vi "ArmTest_LE_and_XZ-AUTO.vi"() -> ()   [LabVIEW 2023]
doc: "Auto test program that coverts RLE to XYZ then to XYZ to RLE"
uses:
  <vilib>/Rock Robotics/WPI/ThirdParty/JAS_Junk/TrajLib/Trajectory_Library.lvlib
panel:
  out "Passed":bool
  out "Extend 2":dbl
  out "Lift 2":dbl
  out "z":dbl
  out "x":dbl
  out "Lift":dbl
  out "Extend":dbl
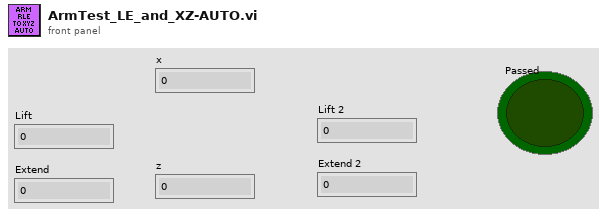
[diagram p1: front panel]
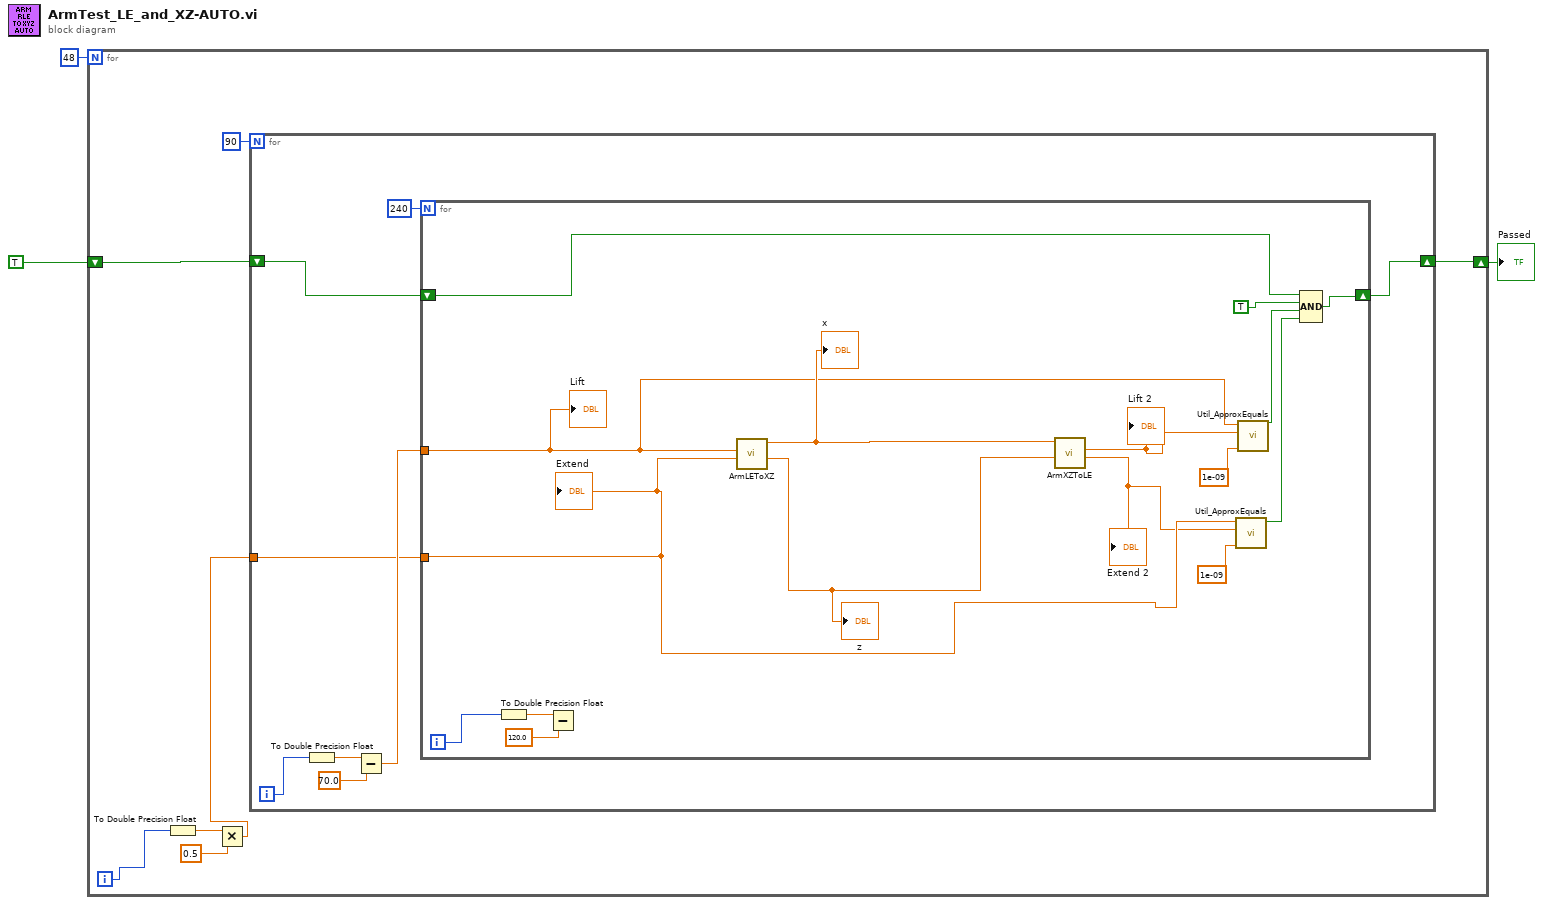
[diagram p0: block diagram]
diagram:
  n1 = for {
    N: 48 -> [_]
    shift-right: [w4] -> w1
    shift-left: TRUE -> [w5]
    i -> [w7]
    n2 = To Double Precision Float(number=w7) -> (double precision float=w9:dbl)
    n3 = Multiply(x=w9, y=0.5) -> (x*y=w6:dbl)
    n4 = for {
      N: 90 -> [_]
      tunnel: w6 -> [w13]
      shift-right: [w11] -> w4
      shift-left: w5 -> [w12]
      i -> [w15]
      n5 = To Double Precision Float(number=w15) -> (double precision float=w17:dbl)
      n6 = Subtract(x=w17, y=70.0) -> (x-y=w14:dbl)
      n7 = for {
        N: 240 -> [_]
        tunnel: w14 -> [w27]
        tunnel: w13 -> [w25]
        shift-right: [w20] -> w11
        shift-left: w12 -> [w23]
        i -> [w32]
        n8 = To Double Precision Float(number=w32) -> (double precision float=w31:dbl)
        n9 = Subtract(x=w31, y=120.0) -> ()  [unwired: 1 out]
        n10 = call "ArmLEToXZ.vi"("Extend"=w25, "Lift"=w27) -> ("z"=w33:dbl, "x"=w34:dbl)  [unwired: 8 in]
        "x" <- w34
        "z" <- w33
        n11 = call "ArmXZToLE.vi"("Z"=w33, "X"=w34) -> ("Extend"=w24:dbl, "Lift"=w26:dbl)  [unwired: 8 in]
        "Lift 2" <- w26
        "Extend 2" <- w24
        n12 = call <vilib>:"Util_ApproxEquals.vi"("Tolerance"=1e-09, "Value 2"=w24, "Value 1"=w25) -> ("ApproxEquals"=w21:bool)  [unwired: 8 in]
        n13 = call <vilib>:"Util_ApproxEquals.vi"("Tolerance"=1e-09, "Value 2"=w26, "Value 1"=w27) -> ("ApproxEquals"=w22:bool)  [unwired: 8 in]
        n14 = Compound Arithmetic op=AND(w23, TRUE ("value"), w22, w21) -> (w20:bool)
        "Extend" <- w25
        "Lift" <- w27
      }
    }
  }
  "Passed" <- w1
